vi "from string.vi"(8 "error in":errorcluster, 9 "data":string, 10 "version":string, 11 "TDMS datalogger configuration in":refnum<class "TDMS datalogger configuration.lvclass">) -> (0 "error out":errorcluster, 3 "TDMS datalogger configuration out":refnum<class "TDMS datalogger configuration.lvclass">)   [LabVIEW 2013, in "TDMS datalogger configuration.lvclass"]
doc: "Provides an interface for loading a module configuration from a file or other serialized data source. It is recommended that all children of this class store data in two sets--data required for its own initialization, and any data required for parent initialization--and that each implementation uses the <b>Call Parent Method</b> primitive to de-serialize parent information. As a result, it is expected that every module configuration class calls <b>component configuration.lvclass:From String.vi</b>."
uses:
  TDMS datalogger configuration.lvclass
  <vilib>/NI/Tag Bus Module Framework/channel/TBM channel.lvclass
  <vilib>/NI/Tag Bus Module Framework/module configuration/TBM module configuration.lvclass
  TDMS datalogger configuration.lvclass/TDMS datalogger configuration.ctl
  <vilib>/NI/Configuration Framework/serializable configuration/NISE_CEF_serializable configuration.lvclass
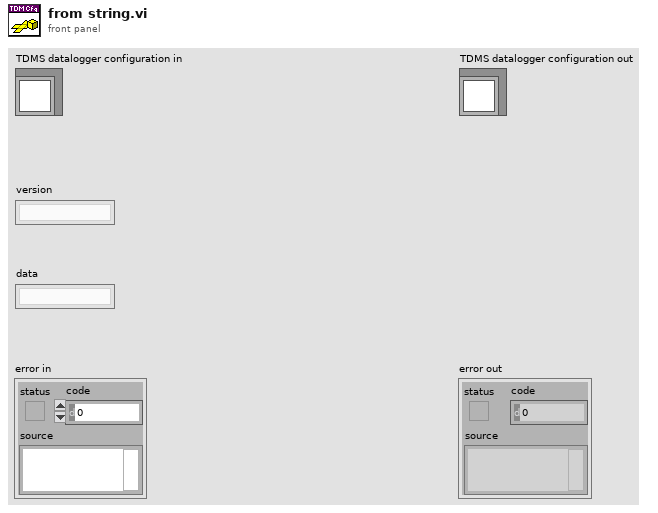
[diagram p1: front panel]
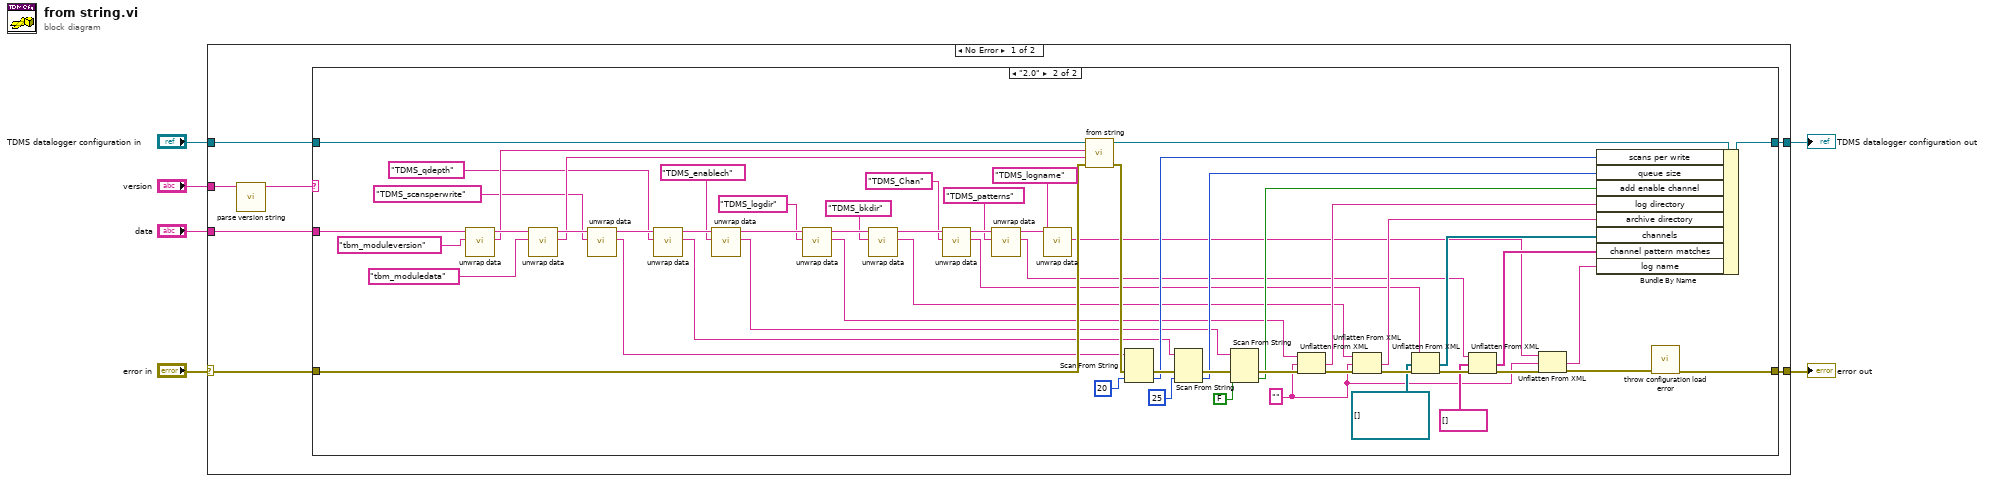
[diagram p0: block diagram]
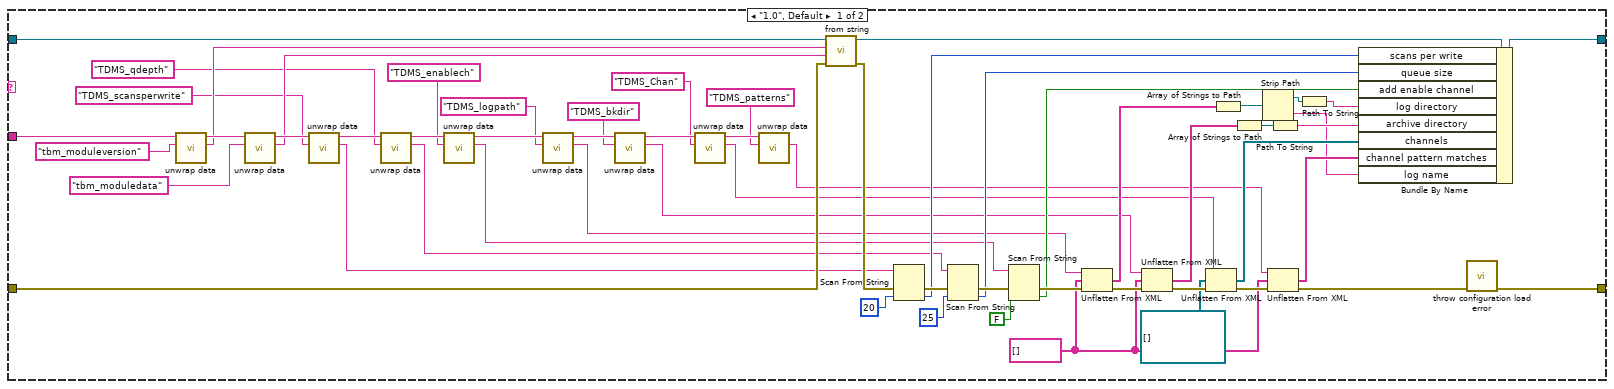
[diagram p2: hidden frame]
diagram:
  n1 = case shown="No Error" "error in" {
    selector: "error in" -> [w7 w131]
    tunnel: "data" -> [w13 _]
    tunnel: "TDMS datalogger configuration in" -> [w12 w130]
    tunnel: [w11 w130] -> w5
    tunnel: [w10 w131] -> w4
    tunnel: "version" -> [w9 _]
    frame No Error {
      n2 = call <vilib>:"parse version string.vi"("full version"=w9) -> ("major.minor version"=w8:string)  [unwired: 7 in, 3 out]
      n3 = case shown="\"2.0\"" w8 {
        tunnel: w13 -> [w54 w112]
        tunnel: w7 -> [w68 w126]
        tunnel: w12 -> [w71 w129]
        tunnel: [w70 w128] -> w11
        tunnel: [w27 w85] -> w10
        frame "1.0", Default {
          w22 = string[] [] ("array of strings")
          n4 = call <vilib>:"unwrap data.vi"("identifier"="tbm_moduleversion" ("additional identifier"), "data to unwrap"=w54) -> ("unwrapped data"=w53:string, "remaining string"=w60:string)  [unwired: 8 in]
          n5 = call <vilib>:"unwrap data.vi"("identifier"="tbm_moduledata" ("additional identifier"), "data to unwrap"=w60) -> ("unwrapped data"=w52:string, "remaining string"=w57:string)  [unwired: 8 in]
          n6 = call <vilib>:"unwrap data.vi"("identifier"="TDMS_scansperwrite" ("additional identifier"), "data to unwrap"=w57) -> ("unwrapped data"=w38:string, "remaining string"=w56:string)  [unwired: 8 in]
          n7 = call <vilib>:"unwrap data.vi"("identifier"="TDMS_qdepth" ("additional identifier"), "data to unwrap"=w56) -> ("unwrapped data"=w36:string, "remaining string"=w55:string)  [unwired: 8 in]
          n8 = call <vilib>:"unwrap data.vi"("identifier"="TDMS_enablech" ("additional identifier"), "data to unwrap"=w55) -> ("unwrapped data"=w34:string, "remaining string"=w42:string)  [unwired: 8 in]
          n9 = call <vilib>:"unwrap data.vi"("identifier"="TDMS_logpath" ("additional identifier"), "data to unwrap"=w42) -> ("unwrapped data"=w32:string, "remaining string"=w41:string)  [unwired: 8 in]
          n10 = call <vilib>:"unwrap data.vi"("identifier"="TDMS_bkdir" ("additional identifier"), "data to unwrap"=w41) -> ("unwrapped data"=w31:string, "remaining string"=w40:string)  [unwired: 8 in]
          n11 = call <vilib>:"unwrap data.vi"("identifier"="TDMS_Chan" ("additional identifier"), "data to unwrap"=w40) -> ("unwrapped data"=w30:string, "remaining string"=w26:string)  [unwired: 8 in]
          n12 = call <vilib>:"unwrap data.vi"("identifier"="TDMS_patterns", "data to unwrap"=w26) -> ("unwrapped data"=w21:string)  [unwired: 8 in, 1 out]
          n13 = call-parent "from string.vi"("error in"=w68, "data"=w52, "version"=w53, "module configuration in"=w71) -> ("error out"=w69:errorcluster, "module configuration out"=w67:refnum<class "TDMS datalogger configuration.lvclass">)  [unwired: 6 in]
          n14 = Scan From String(input string=w38, error in=w69, default 1=u16 20 ("scans per write")) -> (error out=w49:errorcluster, output 1=w43:u16)  [unwired: 2 in, 2 out]
          n15 = Scan From String(input string=w36, error in=w49, default 1=u16 25 ("queue size")) -> (error out=w50:errorcluster, output 1=w45:u16)  [unwired: 2 in, 2 out]
          n16 = Scan From String(input string=w34, error in=w50, default 1=FALSE ("add enable channel")) -> (error out=w51:errorcluster, output 1=w47:bool)  [unwired: 2 in, 2 out]
          n17 = Unflatten From XML(xml string=w32, type=w22, error in (no error)=w51) -> (value=w61:string[], error out=w65:errorcluster)
          n18 = Unflatten From XML(xml string=w31, type=w22, error in (no error)=w65) -> (value=w62:string[], error out=w66:errorcluster)
          n19 = Unflatten From XML(xml string=w30, type=refnum<class "TBM channel.lvclass">[] [] ("channels"), error in (no error)=w66) -> (value=w63:refnum<class "TBM channel.lvclass">[], error out=w24:errorcluster)
          n20 = Array of Strings to Path(0:w61) -> (2:w17:path)  [unwired: 1 in]
          n21 = Array of Strings to Path(0:w62) -> (2:w19:path)  [unwired: 1 in]
          n22 = Strip Path(path=w17) -> (stripped path=w15:path, name=w16:string)
          n23 = Unflatten From XML(xml string=w21, type=w22, error in (no error)=w24) -> (value=w20:string[], error out=w23:errorcluster)
          n24 = Path To String(path=w19) -> (string=w18:string)
          n25 = Path To String(path=w15) -> (string=w14:string)
          n26 = Bundle By Name(cluster=w67, "scans per write"=w43, "queue size"=w45, "add enable channel"=w47, "log directory"=w14, "archive directory"=w18, "channels"=w63, "channel pattern matches"=w20, "log name"=w16) -> (w70:refnum<class "TDMS datalogger configuration.lvclass">)
          n27 = call <vilib>:"throw configuration load error.vi"("error in"=w23) -> ("error out"=w27:errorcluster)  [unwired: 10 in]
        }
        frame "2.0" {
          w76 = ""
          n28 = call <vilib>:"unwrap data.vi"("identifier"="tbm_moduleversion" ("additional identifier"), "data to unwrap"=w112) -> ("unwrapped data"=w111:string, "remaining string"=w118:string)  [unwired: 8 in]
          n29 = call <vilib>:"unwrap data.vi"("identifier"="tbm_moduledata" ("additional identifier"), "data to unwrap"=w118) -> ("unwrapped data"=w110:string, "remaining string"=w115:string)  [unwired: 8 in]
          n30 = call <vilib>:"unwrap data.vi"("identifier"="TDMS_scansperwrite" ("additional identifier"), "data to unwrap"=w115) -> ("unwrapped data"=w96:string, "remaining string"=w114:string)  [unwired: 8 in]
          n31 = call <vilib>:"unwrap data.vi"("identifier"="TDMS_qdepth" ("additional identifier"), "data to unwrap"=w114) -> ("unwrapped data"=w94:string, "remaining string"=w113:string)  [unwired: 8 in]
          n32 = call <vilib>:"unwrap data.vi"("identifier"="TDMS_enablech" ("additional identifier"), "data to unwrap"=w113) -> ("unwrapped data"=w92:string, "remaining string"=w100:string)  [unwired: 8 in]
          n33 = call <vilib>:"unwrap data.vi"("identifier"="TDMS_logdir" ("additional identifier"), "data to unwrap"=w100) -> ("unwrapped data"=w90:string, "remaining string"=w99:string)  [unwired: 8 in]
          n34 = call <vilib>:"unwrap data.vi"("identifier"="TDMS_bkdir" ("additional identifier"), "data to unwrap"=w99) -> ("unwrapped data"=w89:string, "remaining string"=w98:string)  [unwired: 8 in]
          n35 = call <vilib>:"unwrap data.vi"("identifier"="TDMS_Chan" ("additional identifier"), "data to unwrap"=w98) -> ("unwrapped data"=w88:string, "remaining string"=w84:string)  [unwired: 8 in]
          n36 = call <vilib>:"unwrap data.vi"("identifier"="TDMS_patterns", "data to unwrap"=w84) -> ("unwrapped data"=w80:string, "remaining string"=w74:string)  [unwired: 8 in]
          n37 = call <vilib>:"unwrap data.vi"("identifier"="TDMS_logname", "data to unwrap"=w74) -> ("unwrapped data"=w73:string)  [unwired: 8 in, 1 out]
          n38 = call-parent "from string.vi"("error in"=w126, "data"=w110, "version"=w111, "module configuration in"=w129) -> ("error out"=w127:errorcluster, "module configuration out"=w125:refnum<class "TDMS datalogger configuration.lvclass">)  [unwired: 6 in]
          n39 = Scan From String(input string=w96, error in=w127, default 1=u16 20 ("scans per write")) -> (error out=w107:errorcluster, output 1=w101:u16)  [unwired: 2 in, 2 out]
          n40 = Scan From String(input string=w94, error in=w107, default 1=u16 25 ("queue size")) -> (error out=w108:errorcluster, output 1=w103:u16)  [unwired: 2 in, 2 out]
          n41 = Scan From String(input string=w92, error in=w108, default 1=FALSE ("add enable channel")) -> (error out=w109:errorcluster, output 1=w105:bool)  [unwired: 2 in, 2 out]
          n42 = Unflatten From XML(xml string=w90, type=w76, error in (no error)=w109) -> (value=w119:string, error out=w123:errorcluster)
          n43 = Unflatten From XML(xml string=w89, type=w76, error in (no error)=w123) -> (value=w120:string, error out=w124:errorcluster)
          n44 = Unflatten From XML(xml string=w88, type=refnum<class "TBM channel.lvclass">[] [] ("channels"), error in (no error)=w124) -> (value=w121:refnum<class "TBM channel.lvclass">[], error out=w82:errorcluster)
          n45 = Unflatten From XML(xml string=w80, type=string[] [] ("array of strings"), error in (no error)=w82) -> (value=w79:string[], error out=w78:errorcluster)
          n46 = Unflatten From XML(xml string=w73, type=w76, error in (no error)=w78) -> (value=w75:string, error out=w77:errorcluster)
          n47 = Bundle By Name(cluster=w125, "scans per write"=w101, "queue size"=w103, "add enable channel"=w105, "log directory"=w119, "archive directory"=w120, "channels"=w121, "channel pattern matches"=w79, "log name"=w75) -> (w128:refnum<class "TDMS datalogger configuration.lvclass">)
          n48 = call <vilib>:"throw configuration load error.vi"("error in"=w77) -> ("error out"=w85:errorcluster)  [unwired: 10 in]
        }
      }
    }
    frame Error {
    }
  }
  "error out" <- w4
  "TDMS datalogger configuration out" <- w5
